vi "Config Type.vi"(11 "Transition in":refnum<class "Transition.lvclass">) -> (2 "Config Type":refnum<class "Transition Config.lvclass">)   [LabVIEW 2020, in "VolatusSeq.lvlib" / "Transition.lvclass"]
uses:
  Transition.lvclass
  Transition.lvclass/Transition.ctl
  VolatusSeqConfig/Transition Config/Transition Config.lvclass
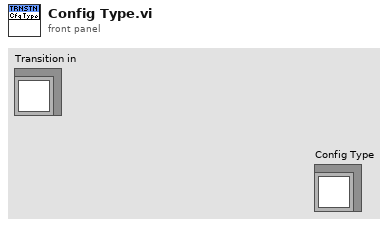
[diagram p1: front panel]
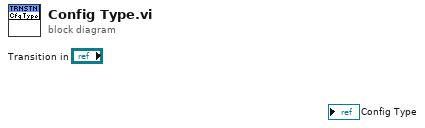
[diagram p0: block diagram]
diagram:
